vi "Process.vi"(0 "reference in":refnum<class "Tester.lvclass">, 5 "error in (no error)":errorcluster) -> (14 "reference out":refnum<class "Tester.lvclass">, 19 "error out":errorcluster)   [LabVIEW 2018, in "Tester.lvclass"]
uses:
  Tester.lvclass
  <vilib>/Utility/miscctls.llb/LVRowAndColumnUnsignedTypeDef.ctl
  controls/LR Mode.ctl
  Reporter_class/Reporter.lvclass
  BKP-911x Power Supply_class/BKP-911x Power Supply.lvclass
  NI-DAQmx_class/NI-DAQmx.lvclass
  BKP-891 LCR Meter_class/BKP-891 LCR Meter.lvclass
panel:
  out "Step Number":i32
  in  "Load Test":bool
  in  "Stop Test":bool
  in  "Start Test":bool
  out "Loaded Test Profile Path":path
  out "Loaded Test Profile":i32(listbox)
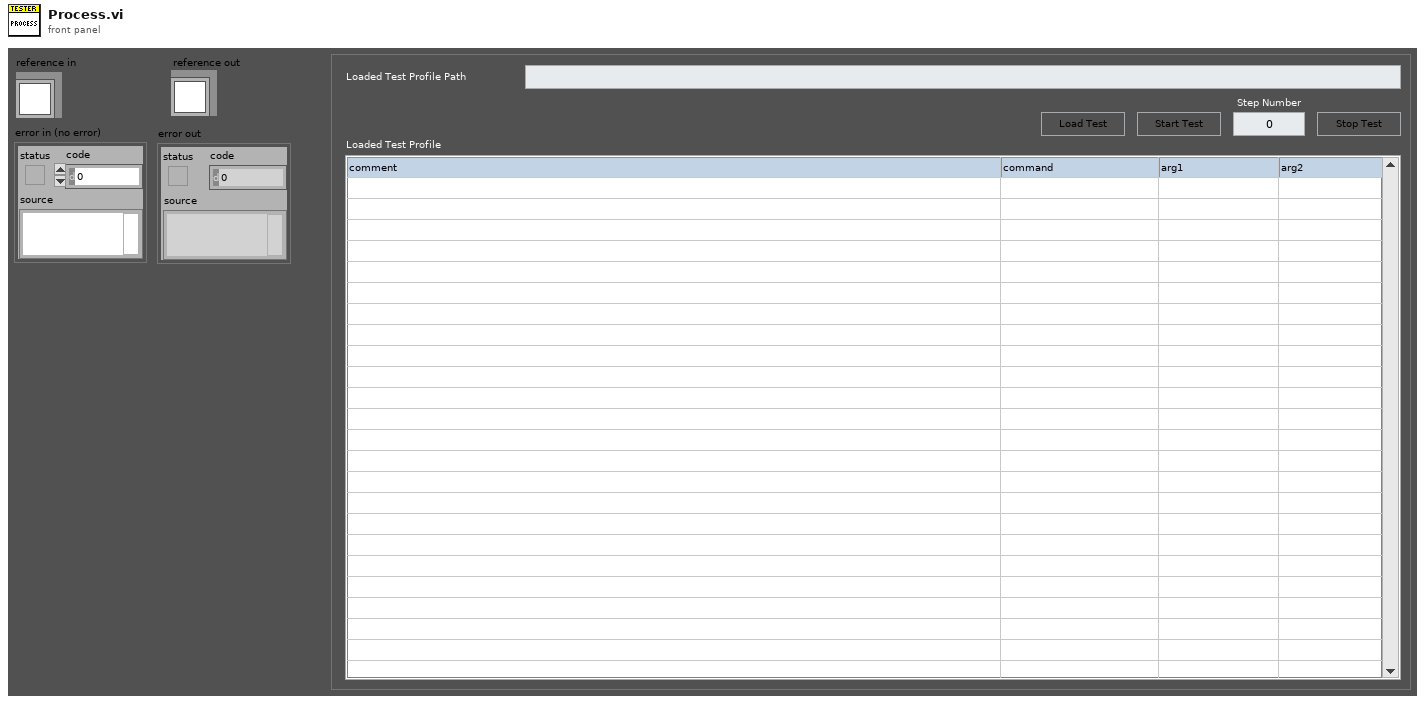
[diagram p1: front panel]
types:
  T1 = cluster{"Event":refnum<event-registration>, "Command":string, "Data":variant, "Testing?":bool, "Loaded Test Steps":string[][], "Args":variant, "Test Step Index":i32, "Step Comment":string}
  T2 = enum8{"Enabled", "Disabled", "Disabled and Grayed Out"}
  T3 = typedef "LVRowAndColumnUnsignedTypeDef.ctl" = cluster{"Row":u32, "Column":u32}
  T4 = typedef "LR Mode.ctl" = enum16{"R - Resistance", "L - Inductance"}
  T5 = typedef "Tester.lvclass/ObjectAttributes.ctl" = cluster{"LCR":refnum<class "BKP-891 LCR Meter.lvclass">, "PSU":refnum<class "BKP-911x Power Supply.lvclass">, "NI-DAQmx":refnum<class "NI-DAQmx.lvclass">, "Reporter":refnum<class "Reporter.lvclass">}
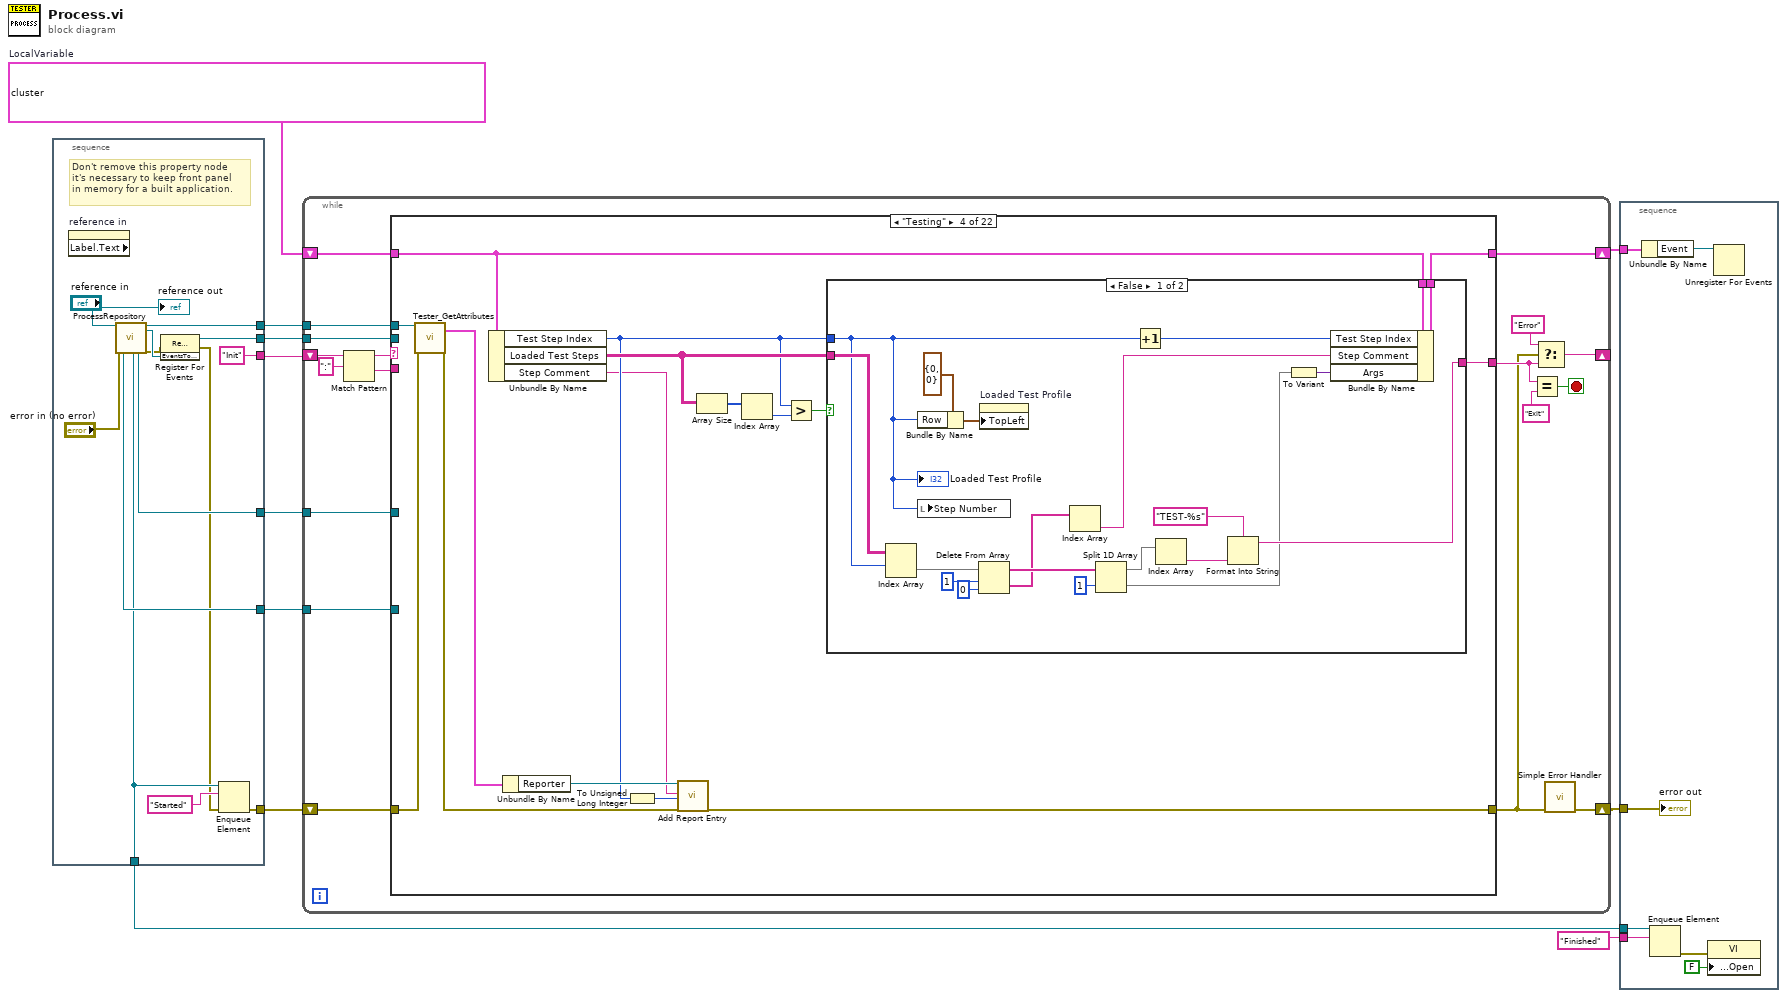
[diagram p0: block diagram]
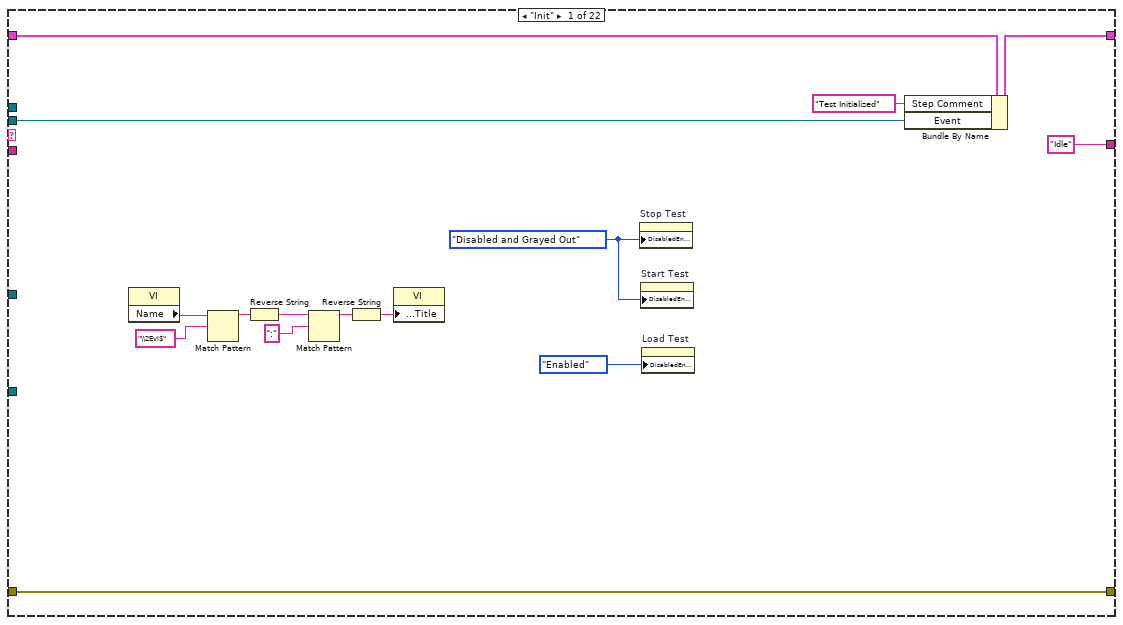
[diagram p2: hidden frame]
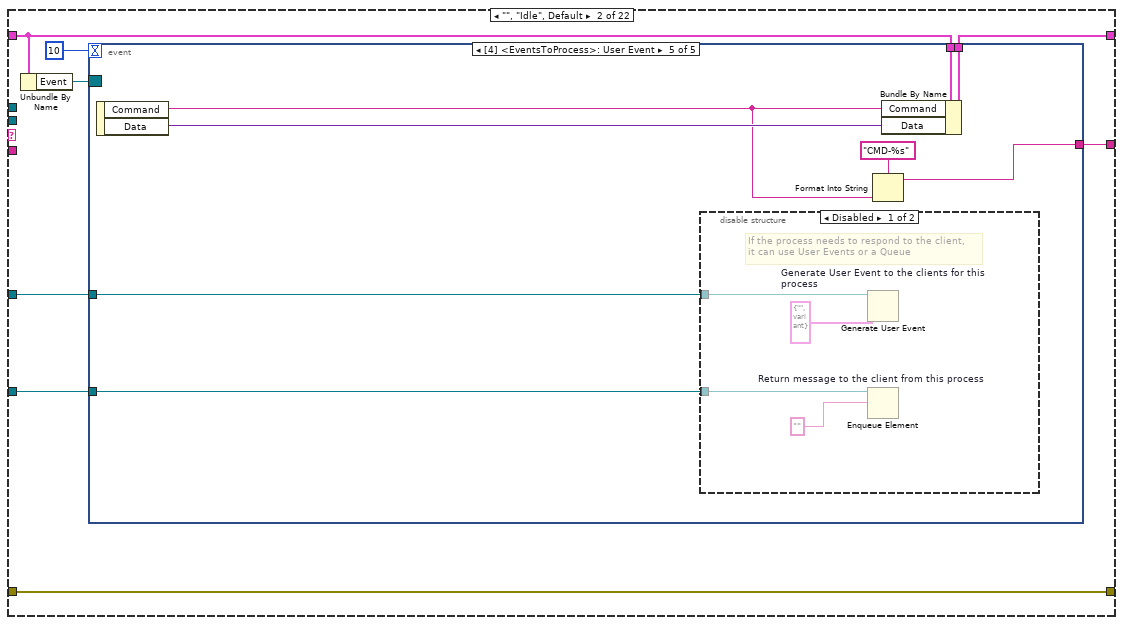
[diagram p3: hidden frame]
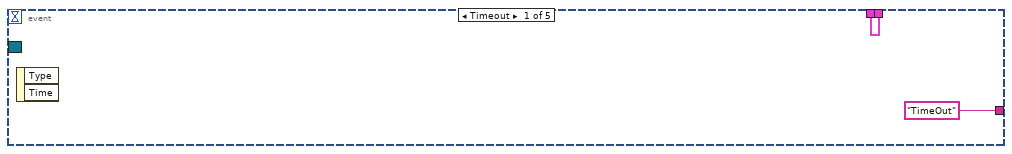
[diagram p4: hidden frame]
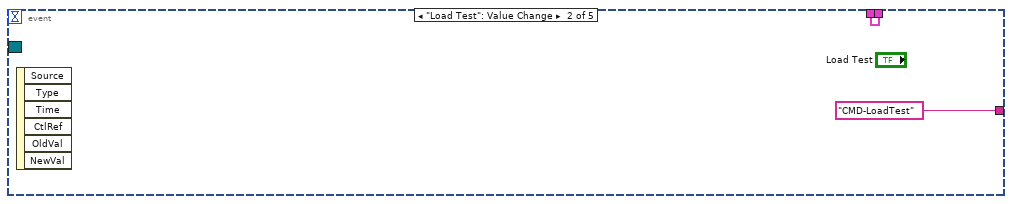
[diagram p5: hidden frame]
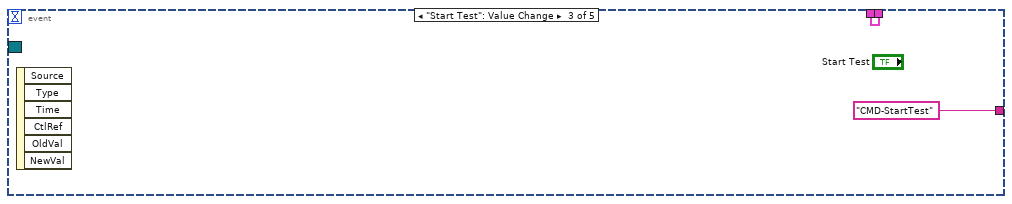
[diagram p6: hidden frame]
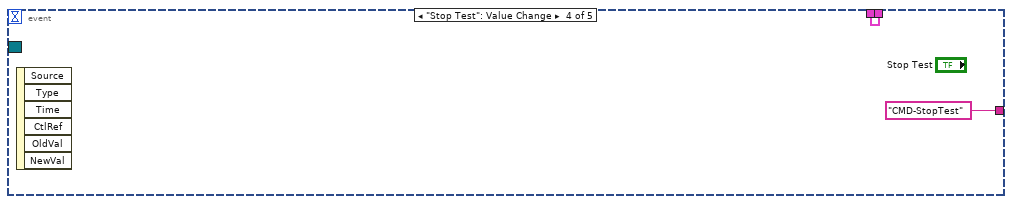
[diagram p7: hidden frame]
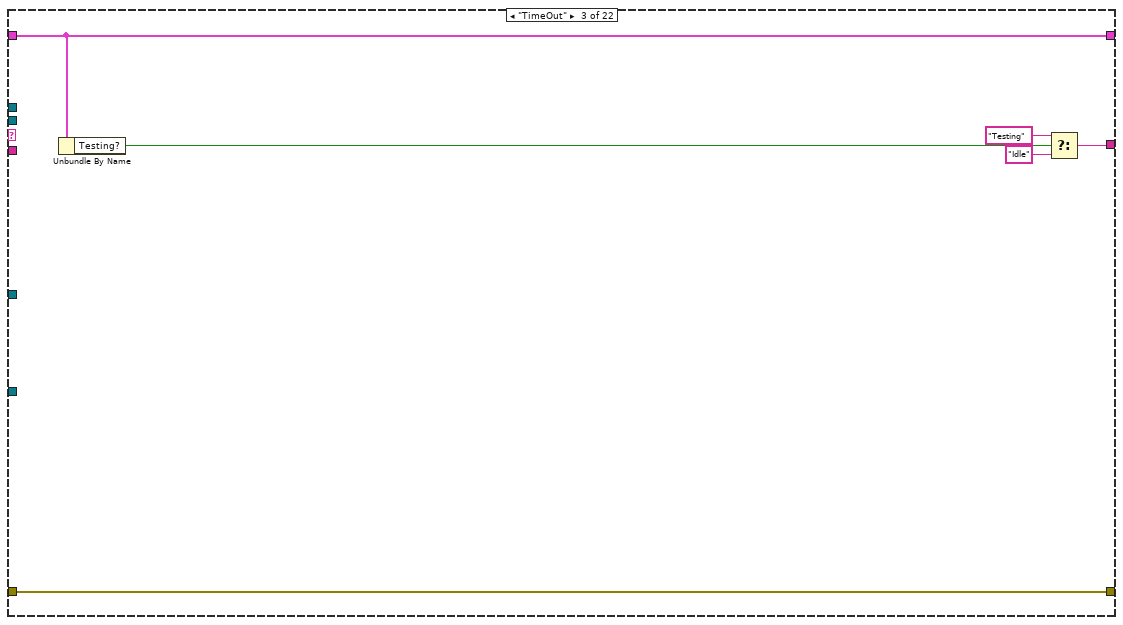
[diagram p9: hidden frame]
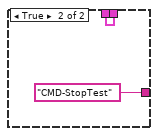
[diagram p10: hidden frame]
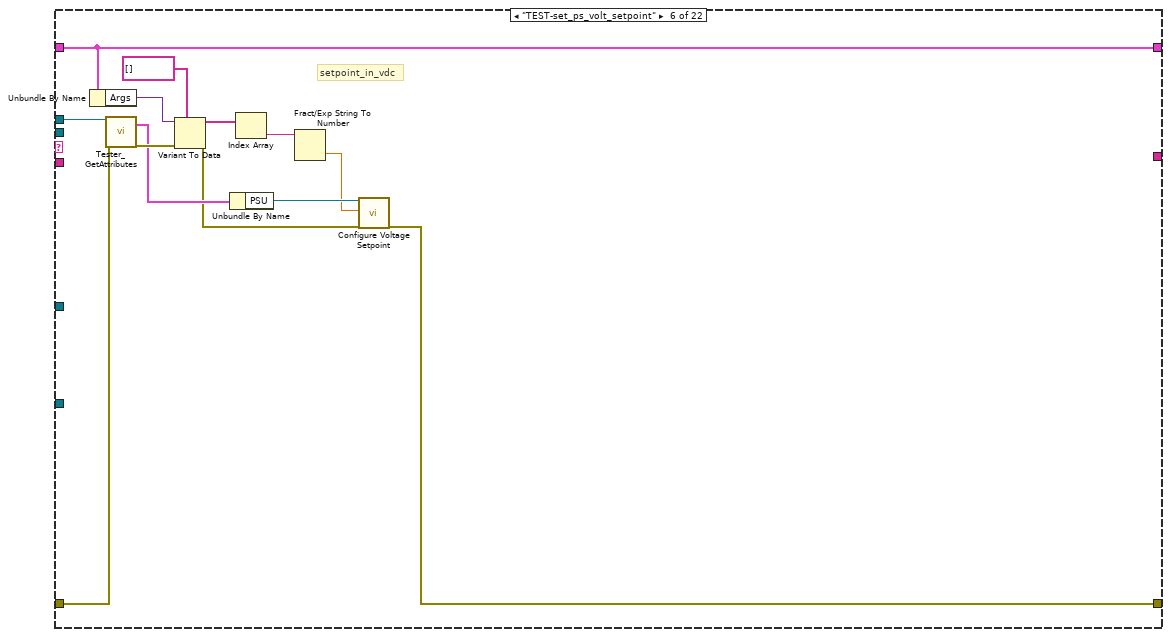
[diagram p12: hidden frame]
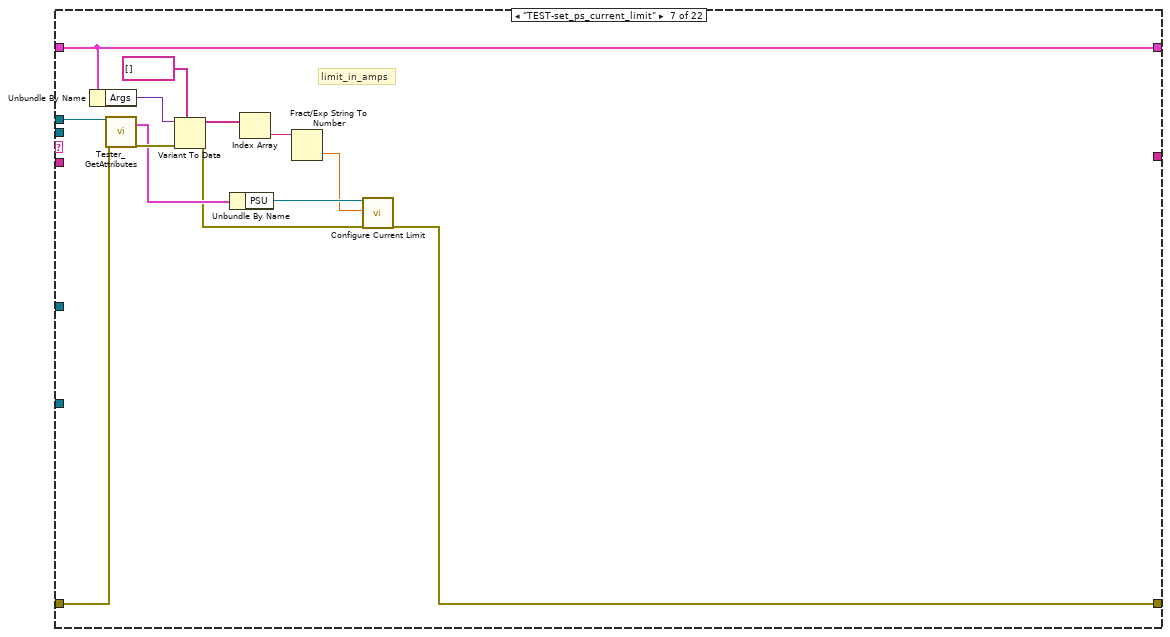
[diagram p13: hidden frame]
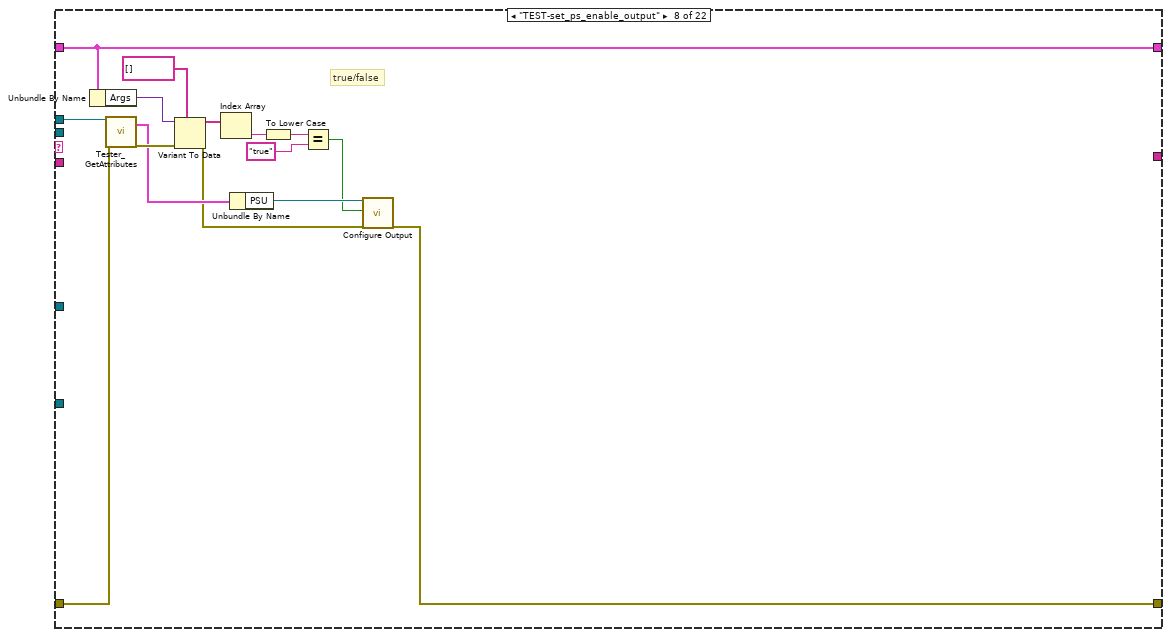
[diagram p14: hidden frame]
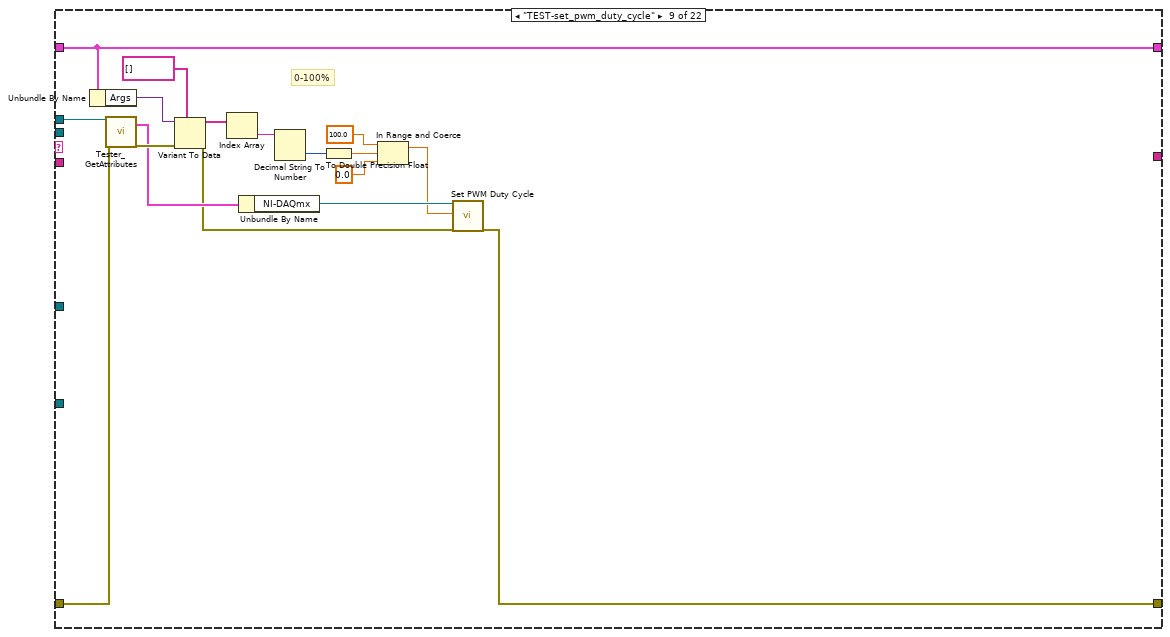
[diagram p15: hidden frame]
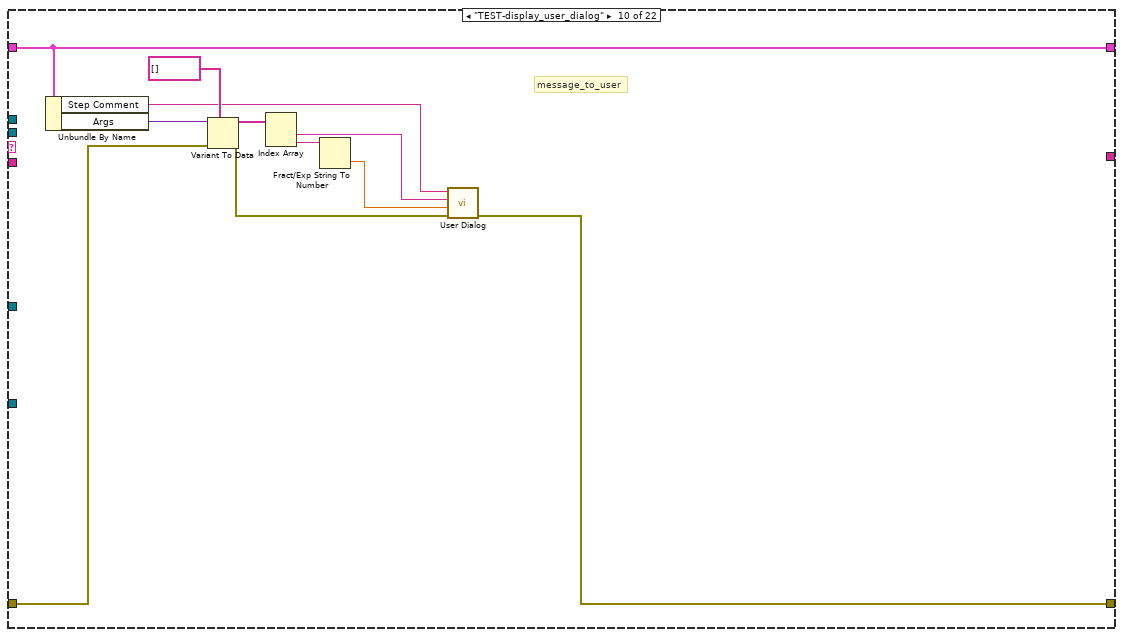
[diagram p16: hidden frame]
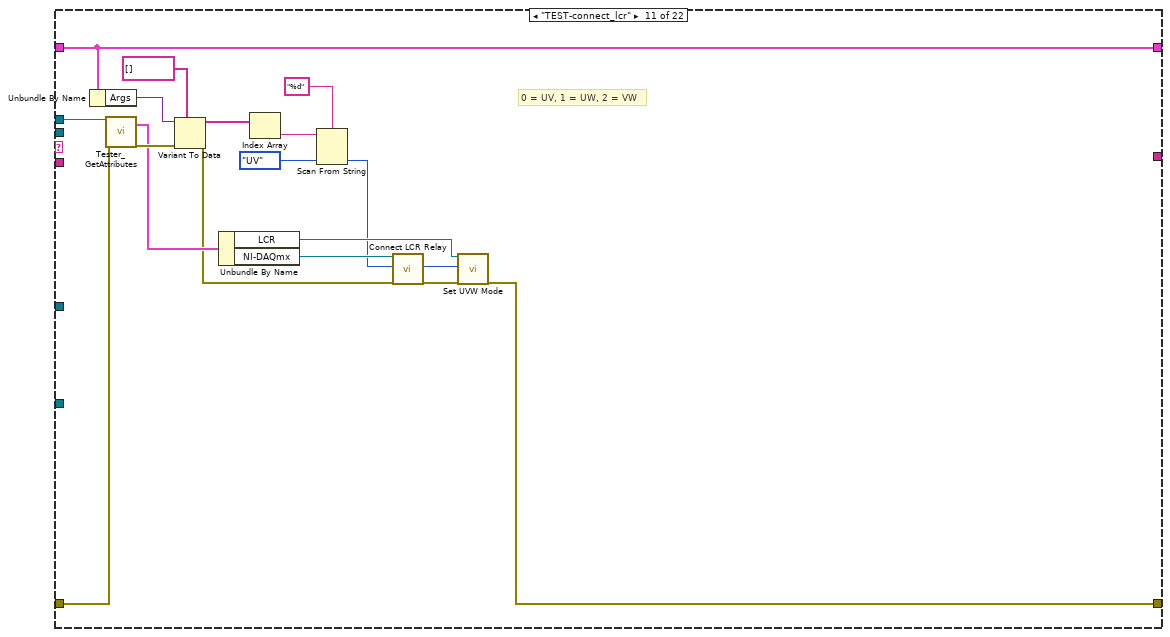
[diagram p17: hidden frame]
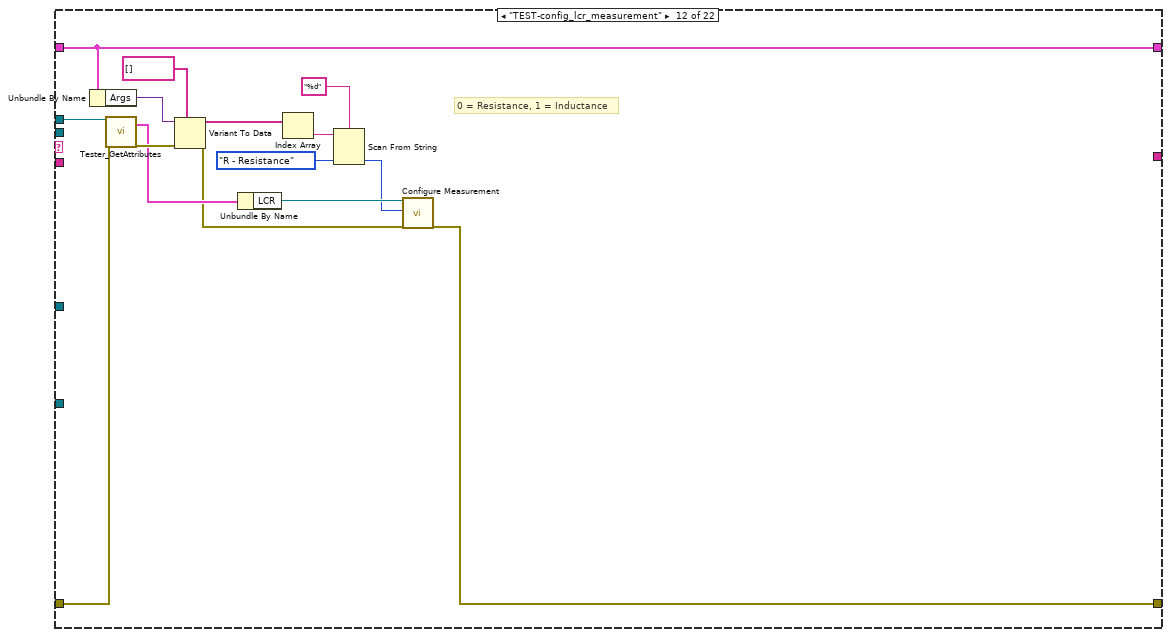
[diagram p18: hidden frame]
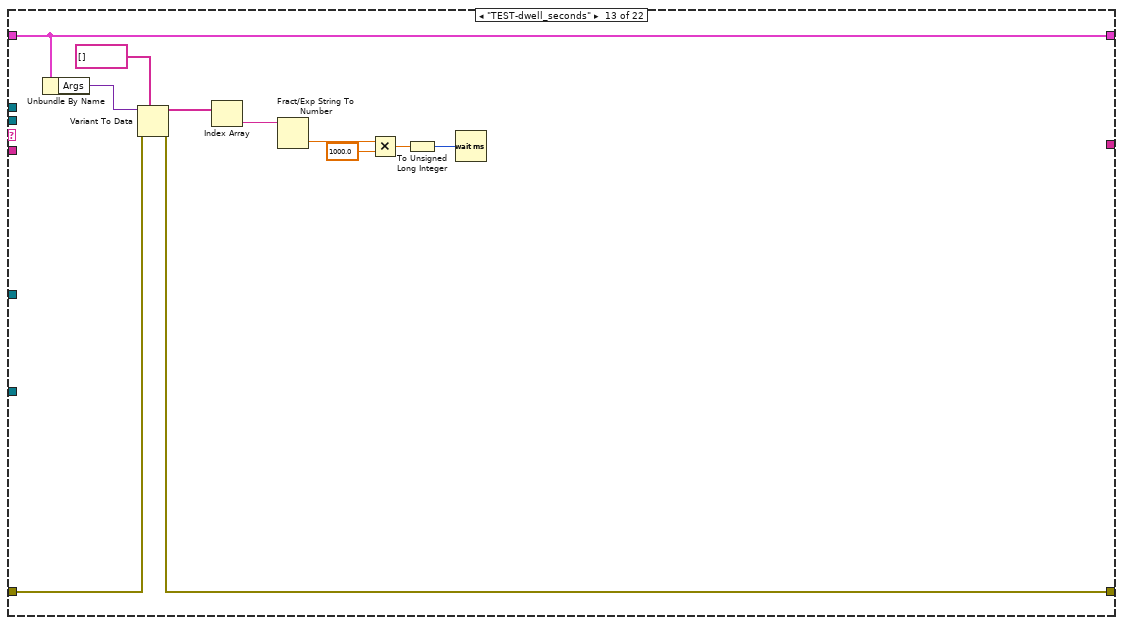
[diagram p19: hidden frame]
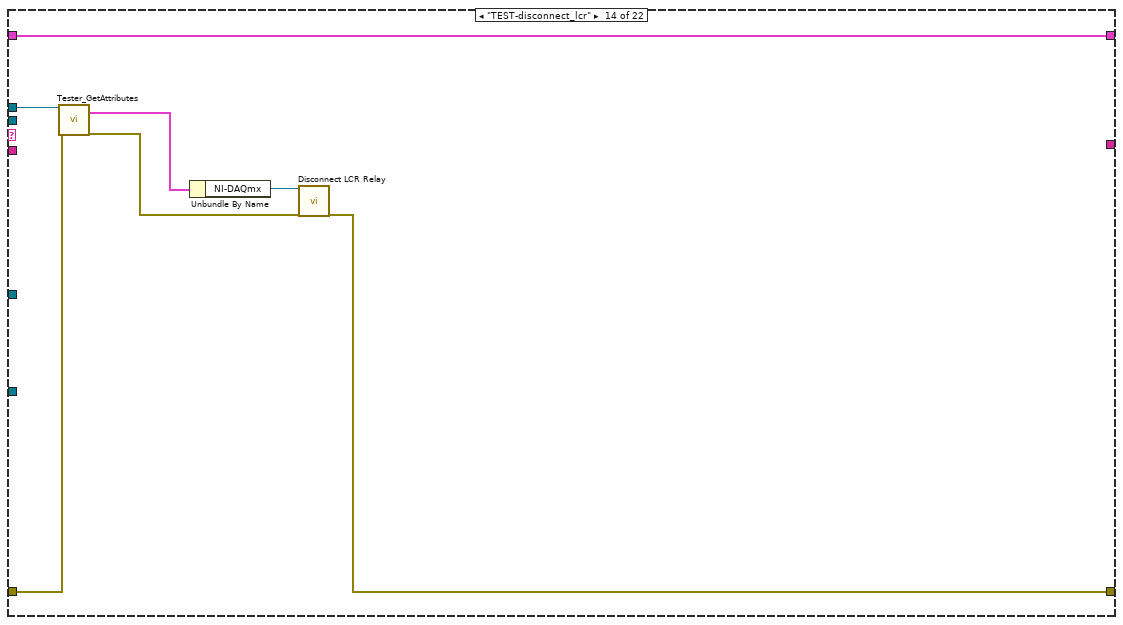
[diagram p20: hidden frame]
diagram:
  w1 = T1 {"Event"=refnum, "Command"="", "Data"=variant, "Testing?"=FALSE, "Loaded Test Steps"=[], "Args"=variant, "Test Step Index"=0, "Step Comment"=""}  # LocalVariable
  n1 = stacked-sequence {
    tunnel: [w17] -> w11
    tunnel: [w24] -> w9
    tunnel: [w14] -> w8
    tunnel: [w18] -> w7
    tunnel: ["Init"] -> w6
    tunnel: [w20] -> w4
    tunnel: [w19] -> w3
    frame #0 {
      # "Don't remove this property node\nit's necessary to keep front panel\nin memory for a built application."
      n2 = property on="reference in" class="LVClassControl (strict)" props=["Label", "Text"]() -> ()  [unwired: 2 in, 3 out]
      n3 = call "ProcessRepository.vi"("reference in"="reference in", "error in (no error)"="error in (no error)") -> ("QueueFromProcess"=w19:refnum<queue>, "ProcessSyncQueue"=w18:refnum<queue>, "EventFromProcess"=w20:refnum<user-event>, "reference out"=w24:refnum<class "Tester.lvclass">, "EventsToProcess"=w15:refnum<user-event>, "error out"=w13:errorcluster)  [unwired: 10 in, 2 out]
      n4 = register-events(error in=w13, w15) -> (reference out=w14:refnum<event-registration>, error out=w12:errorcluster)  [unwired: 1 in]
      n5 = Enqueue Element(queue=w18, element="Started", error in (no error)=w12) -> (error out=w17:errorcluster)  [unwired: 1 in, 2 out]
      "reference out" <- "reference in"
    }
  }
  n6 = while {
    shift-right: [w25] -> w10
    shift-left: w11 -> [w40]
    tunnel: w9 -> [w41]
    tunnel: w8 -> [w42]
    shift-right: [w34] -> _
    shift-left: w6 -> [w38]
    shift-right: [w30] -> w5
    shift-left: w1 -> [w29]
    tunnel: w4 -> [w28]
    tunnel: w3 -> [w27]
    stop <- w31 stop-if-true
    n7 = Match Pattern(string=w38, regular expression=":") -> (before substring=w37:string, after substring=w36:string)  [unwired: 1 in, 2 out]
    n8 = case shown="\"Testing\"" w37 {
      tunnel: w40 -> [w56 w61 w91 w99 w131 w143 w156 w171 w188 w200 w216 w231 w243 w249 w256 w259 w261 _ w306 w331 w350 w353]
      tunnel: [w56 w61 w91 w95 w131 w132 w145 w160 w180 w193 w203 w221 w238 w244 w251 w259 w261 w262 w301 w330 w350 w353] -> w26
      tunnel: w42 -> [w47 _ _ _ _ _ _ _ _ _ _ _ _ _ _ _ _ _ _ _ _ _]
      tunnel: w41 -> [_ _ _ w100 _ w144 w157 w172 w189 _ w217 w232 _ w250 w257 _ _ _ w305 w332 _ _]
      tunnel: w36 -> [_ _ _ _ _ _ _ _ _ _ _ _ _ _ _ _ _ _ _ _ _ _]
      tunnel: ["Idle" ("t") w65 w86 w105 _ _ _ _ _ _ _ _ _ _ _ _ _ _ w315 w335 _ "Exit" ("y")] -> w33
      tunnel: [w57 w64 w90 w106 w130 w142 w155 w170 w187 w199 w215 w230 w242 w248 w255 w258 w260 w263 w314 w336 w349 w351] -> w30
      tunnel: w29 -> [w46 w58 w90 w107 w130 w142 w155 w170 w187 w199 w215 w230 w242 w248 w255 w258 w260 w264 w313 w334 w349 w351]
      tunnel: w28 -> [_ w60 _ _ _ _ _ _ _ _ _ _ _ _ _ _ _ _ _ _ _ _]
      tunnel: w27 -> [_ w59 _ _ _ _ _ _ _ _ _ _ _ _ _ _ _ _ _ _ _ _]
      frame "Init" {
        w44 = T2."Disabled and Grayed Out" ("Disabled")
        n9 = property class="VI"() -> ("Name"=w54:string)  [unwired: 2 in, 2 out]
        n10 = Match Pattern(string=w54, regular expression="\\2Evi$") -> (before substring=w52:string)  [unwired: 1 in, 3 out]
        n11 = Reverse String(1:w52) -> (0:w51:string)
        n12 = Match Pattern(string=w51, regular expression=":") -> (before substring=w49:string)  [unwired: 1 in, 3 out]
        n13 = Reverse String(1:w49) -> (0:w48:string)
        n14 = property class="VI"("Front Panel.Title"=w48) -> ()  [unwired: 2 in, 2 out]
        n15 = property on="Stop Test" class="Bool"("DisabledEnum"=w44) -> ()  [unwired: 2 in, 2 out]
        n16 = property on="Start Test" class="Bool"("DisabledEnum"=w44) -> ()  [unwired: 2 in, 2 out]
        n17 = property on="Load Test" class="Bool"("DisabledEnum"=T2."Enabled" ("Disabled")) -> ()  [unwired: 2 in, 2 out]
        n18 = Bundle By Name(cluster=w46, "Step Comment"="Test Initialized", "Event"=w47) -> (w57:T1)
      }
      frame "", "Idle", Default {
        n19 = Unbundle By Name(w58) -> ("Event"=w63:refnum<event-registration>)
        n20 = event shown="[4] <EventsToProcess>: User Event" {
          selector: w63 -> [_ _ _ _ _]
          dyn-events: _ -> [_ _ _ _ _]
          timeout: 10 -> [_ _ _ _ _]
          tunnel: ["TimeOut" ("t") "CMD-LoadTest" ("t") "CMD-StartTest" ("t") "CMD-StopTest" ("t") w77] -> w65
          tunnel: w58 -> [w66 w69 w71 w73 w81]
          tunnel: [w66 w69 w71 w73 w80] -> w64
          tunnel: w60 -> [_ _ _ _ w75]
          tunnel: w59 -> [_ _ _ _ w74]
          event Timeout {
            n21 = event-data() -> ()  [unwired: 1 in, 2 out]
          }
          event "Load Test": Value Change {
            n22 = event-data() -> ()  [unwired: 1 in, 6 out]
          }
          event "Start Test": Value Change {
            n23 = event-data() -> ()  [unwired: 1 in, 6 out]
          }
          event "Stop Test": Value Change {
            n24 = event-data() -> ()  [unwired: 1 in, 6 out]
          }
          event User Event {
            n25 = event-data() -> ("Command"=w76:string, "Data"=w79:variant)  [unwired: 1 in]
            n26 = disable-structure shown="Disabled" {
              disable-tunnel: w75 -> [w85 _]
              disable-tunnel: w74 -> [w84 _]
              frame Disabled {
                # "If the process needs to respond to the client,\nit can use User Events or a Queue"
                n27 = Generate User Event "Generate User Event to the clients for this process"(user event=w85, event data cluster=cluster{"Command":string, "Data":variant} {"Command"="", "Data"=variant} ("event data")) -> ()  [unwired: 2 in, 2 out]
                n28 = Enqueue Element "Return message to the client from this process"(queue=w84, element="") -> ()  [unwired: 2 in, 3 out]
              }
              frame Enabled {
              }
            }
            n29 = Format Into String(format string="CMD-%s", w76) -> (resulting string=w77:string)  [unwired: 2 in, 1 out]
            n30 = Bundle By Name(cluster=w81, "Command"=w76, "Data"=w79) -> (w80:T1)
          }
        }
      }
      frame "TimeOut" {
        n31 = Unbundle By Name(w90) -> ("Testing?"=w89:bool)
        n32 = Select(t="Testing", s=w89, f="Idle" ("t")) -> (s? t:f=w86:string)
      }
      frame "Testing" {
        n33 = call "Tester_GetAttributes.vi"("reference in"=w100, "error in (no error)"=w99) -> ("Data"=w98:T5, "error out"=w96:errorcluster)  [unwired: 14 in, 2 out]
        n34 = Unbundle By Name(w107) -> ("Test Step Index"=w94:i32, "Loaded Test Steps"=w104:string[][], "Step Comment"=w92:string)
        n35 = Unbundle By Name(w98) -> ("Reporter"=w97:refnum<class "Reporter.lvclass">)
        n36 = To Unsigned Long Integer(number=w94) -> (unsigned 32bit integer=w93:u32)
        n37 = call-dynamic "Add Report Entry.vi"("reference in"=w97, "comment"=w92, "step_index"=w93, "error in (no error)"=w96) -> ("error out"=w95:errorcluster)  [unwired: 14 in, 1 out]
        n38 = Array Size(array=w104) -> (size(s)=w103:i32[])
        n39 = Index Array(array=w103) -> (element=w102:i32)  [unwired: 1 in]
        n40 = Greater?(x=w94, y=w102) -> (0:w101:bool)
        n41 = case shown="False" w101 {
          tunnel: w107 -> [w127 w129]
          tunnel: [w126 w129] -> w106
          tunnel: w104 -> [w124 _]
          tunnel: w94 -> [w109 _]
          tunnel: [w115 "CMD-StopTest" ("y")] -> w105
          frame False {
            n42 = Index Array(array=w124, index (row)=w109) -> (element=w123:string[])  [unwired: 1 in]
            n43 = Bundle By Name(cluster=T3 {"Row"=0, "Column"=0} ("Top Left Visible Cell"), "Row"=w109) -> (w108:T3)
            n44 = local write "Step Number"(w109) -> ()
            n45 = Delete From Array(array=w123, length=1, index=0) -> (deleted portion=w112:string[], array with subset deleted=w120:string[])
            n46 = property on="Loaded Test Profile" class="MCListbox (strict)"("TopLeft"=w108) -> ()  [unwired: 2 in, 2 out]
            n47 = Index Array(array=w112) -> (element=w111:string)  [unwired: 1 in]
            n48 = Split 1D Array(array=w120, index=1) -> (first subarray=w118:string[], second subarray=w114:string[])
            n49 = Increment(x=w109) -> (x+1=w125:i32)
            n50 = Index Array(array=w118) -> (element=w116:string)  [unwired: 1 in]
            n51 = Format Into String(format string="TEST-%s", w116) -> (resulting string=w115:string)  [unwired: 2 in, 1 out]
            n52 = To Variant(anything=w114) -> (Variant=w113:variant)
            n53 = Bundle By Name(cluster=w127, "Test Step Index"=w125, "Step Comment"=w111, "Args"=w113) -> (w126:T1)
            "Loaded Test Profile" <- w109
          }
          frame True {
          }
        }
      }
      frame "---- TEST METHODS START ----" {
        # "read arguments from variant in shift register"
      }
      frame "TEST-set_ps_volt_setpoint" {
        # "setpoint_in_vdc"
        n54 = Unbundle By Name(w142) -> ("Args"=w140:variant)
        n55 = call "Tester_GetAttributes.vi"("reference in"=w144, "error in (no error)"=w143) -> ("Data"=w138:T5, "error out"=w141:errorcluster)  [unwired: 14 in, 2 out]
        n56 = Variant To Data(error in=w141, type=string[] [], Variant=w140) -> (data=w137:string[], error out=w133:errorcluster)
        n57 = Unbundle By Name(w138) -> ("PSU"=w135:refnum<class "BKP-911x Power Supply.lvclass">)
        n58 = Index Array(array=w137) -> (element=w136:string)  [unwired: 1 in]
        n59 = Fract/Exp String To Number(string=w136) -> (number=w134:dbl)  [unwired: 3 in, 1 out]
        n60 = call-dynamic "Configure Voltage Setpoint.vi"("reference in"=w135, "Voltage Setpoint (V)"=w134, "error in (no error)"=w133) -> ("error out"=w132:errorcluster)  [unwired: 15 in, 1 out]
      }
      frame "TEST-set_ps_current_limit" {
        # "limit_in_amps"
        n61 = Unbundle By Name(w155) -> ("Args"=w153:variant)
        n62 = call "Tester_GetAttributes.vi"("reference in"=w157, "error in (no error)"=w156) -> ("Data"=w151:T5, "error out"=w154:errorcluster)  [unwired: 14 in, 2 out]
        n63 = Variant To Data(error in=w154, type=string[] [], Variant=w153) -> (data=w150:string[], error out=w146:errorcluster)
        n64 = Unbundle By Name(w151) -> ("PSU"=w148:refnum<class "BKP-911x Power Supply.lvclass">)
        n65 = Index Array(array=w150) -> (element=w149:string)  [unwired: 1 in]
        n66 = Fract/Exp String To Number(string=w149) -> (number=w147:dbl)  [unwired: 3 in, 1 out]
        n67 = call-dynamic "Configure Current Limit.vi"("reference in"=w148, "Current Limit (0.0 A)"=w147, "error in (no error)"=w146) -> ("error out"=w145:errorcluster)  [unwired: 15 in, 1 out]
      }
      frame "TEST-set_ps_enable_output" {
        # "true/false"
        n68 = Unbundle By Name(w170) -> ("Args"=w168:variant)
        n69 = call "Tester_GetAttributes.vi"("reference in"=w172, "error in (no error)"=w171) -> ("Data"=w166:T5, "error out"=w169:errorcluster)  [unwired: 14 in, 2 out]
        n70 = Variant To Data(error in=w169, type=string[] [], Variant=w168) -> (data=w165:string[], error out=w161:errorcluster)
        n71 = Index Array(array=w165) -> (element=w159:string)  [unwired: 1 in]
        n72 = Unbundle By Name(w166) -> ("PSU"=w163:refnum<class "BKP-911x Power Supply.lvclass">)
        n73 = To Lower Case(string=w159) -> (all lower case string=w158:string)
        n74 = Equal?(x=w158, y="true") -> (x = y?=w162:bool)
        n75 = call-dynamic "Configure Output.vi"("reference in"=w163, "Enable Output (T: Enable)"=w162, "error in (no error)"=w161) -> ("error out"=w160:errorcluster)  [unwired: 15 in, 1 out]
      }
      frame "TEST-set_pwm_duty_cycle" {
        # "0-100%"
        n76 = Unbundle By Name(w187) -> ("Args"=w185:variant)
        n77 = call "Tester_GetAttributes.vi"("reference in"=w189, "error in (no error)"=w188) -> ("Data"=w183:T5, "error out"=w186:errorcluster)  [unwired: 14 in, 2 out]
        n78 = Variant To Data(error in=w186, type=string[] [], Variant=w185) -> (data=w179:string[], error out=w181:errorcluster)
        n79 = Index Array(array=w179) -> (element=w178:string)  [unwired: 1 in]
        n80 = Unbundle By Name(w183) -> ("NI-DAQmx"=w182:refnum<class "NI-DAQmx.lvclass">)
        n81 = Decimal String To Number(string=w178) -> (number=w177:i32)  [unwired: 2 in, 1 out]
        n82 = To Double Precision Float(number=w177) -> (double precision float=w176:dbl)
        n83 = In Range and Coerce(upper limit=100.0, x=w176, lower limit=0.0) -> (coerced(x)=w173:dbl)  [unwired: 1 out]
        n84 = call-dynamic "Set PWM Duty Cycle.vi"("reference in"=w182, "PWM Duty Cycle (%)"=w173, "error in (no error)"=w181) -> ("error out"=w180:errorcluster)  [unwired: 15 in, 1 out]
      }
      frame "TEST-display_user_dialog" {
        # "message_to_user"
        n85 = Unbundle By Name(w199) -> ("Step Comment"=w190:string, "Args"=w198:variant)
        n86 = Variant To Data(error in=w200, type=string[] [], Variant=w198) -> (data=w196:string[], error out=w194:errorcluster)
        n87 = Index Array(array=w196) -> (element #1=w195:string, element #2=w192:string)  [unwired: 2 in]
        n88 = Fract/Exp String To Number(string=w192) -> (number=w191:dbl)  [unwired: 3 in, 1 out]
        n89 = call "User Dialog.vi"("error in (no error)"=w194, "Timeout (seconds)"=w191, "Message"=w195, "Title"=w190) -> ("error out"=w193:errorcluster)  [unwired: 7 in]
      }
      frame "TEST-connect_lcr" {
        # "0 = UV, 1 = UW, 2 = VW"
        n90 = Unbundle By Name(w215) -> ("Args"=w213:variant)
        n91 = call "Tester_GetAttributes.vi"("reference in"=w217, "error in (no error)"=w216) -> ("Data"=w211:T5, "error out"=w214:errorcluster)  [unwired: 14 in, 2 out]
        n92 = Variant To Data(error in=w214, type=string[] [], Variant=w213) -> (data=w208:string[], error out=w209:errorcluster)
        n93 = Unbundle By Name(w211) -> ("LCR"=w202:refnum<class "BKP-891 LCR Meter.lvclass">, "NI-DAQmx"=w210:refnum<class "NI-DAQmx.lvclass">)
        n94 = Index Array(array=w208) -> (element=w206:string)  [unwired: 1 in]
        n95 = Scan From String(format string="%d", input string=w206, default 1=enum16{"UV", "UW", "VW"}."UV" ("Relay Mode")) -> (output 1=w201:enum16{"UV", "UW", "VW"})  [unwired: 2 in, 3 out]
        n96 = call-dynamic "Connect LCR Relay.vi"("reference in"=w210, "Relay Mode"=w201, "error in (no error)"=w209) -> ("error out"=w204:errorcluster)  [unwired: 15 in, 1 out]
        n97 = call-dynamic "Set UVW Mode.vi"("reference in"=w202, "UVW Mode"=w201, "error in (no error)"=w204) -> ("error out"=w203:errorcluster)  [unwired: 15 in, 1 out]
      }
      frame "TEST-config_lcr_measurement" {
        # "0 = Resistance, 1 = Inductance"
        n98 = Unbundle By Name(w230) -> ("Args"=w228:variant)
        n99 = call "Tester_GetAttributes.vi"("reference in"=w232, "error in (no error)"=w231) -> ("Data"=w226:T5, "error out"=w229:errorcluster)  [unwired: 14 in, 2 out]
        n100 = Variant To Data(error in=w229, type=string[] [], Variant=w228) -> (data=w225:string[], error out=w222:errorcluster)
        n101 = Unbundle By Name(w226) -> ("LCR"=w220:refnum<class "BKP-891 LCR Meter.lvclass">)
        n102 = Index Array(array=w225) -> (element=w224:string)  [unwired: 1 in]
        n103 = Scan From String(format string="%d", input string=w224, default 1=LR_Mode."R - Resistance" ("LR Mode")) -> (output 1=w218:T4)  [unwired: 2 in, 3 out]
        n104 = call-dynamic "Configure Measurement.vi"("reference in"=w220, "LR Mode"=w218, "error in (no error)"=w222) -> ("error out"=w221:errorcluster)  [unwired: 15 in, 1 out]
      }
      frame "TEST-dwell_seconds" {
        n105 = Unbundle By Name(w242) -> ("Args"=w241:variant)
        n106 = Variant To Data(error in=w243, type=string[] [], Variant=w241) -> (data=w239:string[], error out=w238:errorcluster)
        n107 = Index Array(array=w239) -> (element=w237:string)  [unwired: 1 in]
        n108 = Fract/Exp String To Number(string=w237) -> (number=w236:dbl)  [unwired: 3 in, 1 out]
        n109 = Multiply(x=w236, y=1000.0) -> (x*y=w234:dbl)
        n110 = To Unsigned Long Integer(number=w234) -> (unsigned 32bit integer=w233:u32)
        n111 = Wait (ms)(milliseconds to wait=w233) -> ()  [unwired: 1 out]
      }
      frame "TEST-disconnect_lcr" {
        n112 = call "Tester_GetAttributes.vi"("reference in"=w250, "error in (no error)"=w249) -> ("Data"=w247:T5, "error out"=w245:errorcluster)  [unwired: 14 in, 2 out]
        n113 = Unbundle By Name(w247) -> ("NI-DAQmx"=w246:refnum<class "NI-DAQmx.lvclass">)
        n114 = call-dynamic "Disconnect LCR Relay.vi"("reference in"=w246, "error in (no error)"=w245) -> ("error out"=w244:errorcluster)  [unwired: 16 in, 1 out]
      }
      frame "TEST-tare_lcr" {
        n115 = call "Tester_GetAttributes.vi"("reference in"=w257, "error in (no error)"=w256) -> ("Data"=w254:T5, "error out"=w252:errorcluster)  [unwired: 14 in, 2 out]
        n116 = Unbundle By Name(w254) -> ("LCR"=w253:refnum<class "BKP-891 LCR Meter.lvclass">)
        n117 = call-dynamic "Set Tare Offset.vi"("reference in"=w253, "error in (no error)"=w252) -> ("error out"=w251:errorcluster)  [unwired: 16 in, 1 out]
      }
      frame "---- TEST METHODS END ----" {
      }
      frame "---- COMMANDS START----" {
      }
      frame "CMD-LoadTest" {
        n118 = call "Get File Paths.vi"() -> ("Test Profiles Directory"=w273:path)  [unwired: 10 in, 1 out]
        n119 = call "File Dialog"("start path"=w273, "prompt"="Select a test profile (csv) to load...", "button label"="Load Test", "pattern (all files)"="*.csv", "pattern label"="Comma Separated Values") -> ("selected path"=w267:path, "cancelled"=w268:bool, "error out"=w266:errorcluster)  [unwired: 7 in, 1 out]
        n120 = call <vilib>:"Clear Errors.vi"("error in (no error)"=w266) -> ("error out"=w265:errorcluster)  [unwired: 5 in, 1 out]
        n121 = case shown="False" w268 {
          tunnel: w267 -> [w295 _]
          tunnel: w265 -> [w296 w299]
          tunnel: w264 -> [w298 w300]
          tunnel: [w297 w300] -> w263
          tunnel: [w277 w299] -> w262
          frame False {
            # "remove header row"
            n122 = Open/Create/Replace File(file path (use dialog)=w295, error in=w296, access (0:read/write)=enum16{"read/write", "read-only", "write-only"}."read-only") -> (refnum out=w293:refnum<file>, error out=w292:errorcluster)  [unwired: 3 in, 1 out]
            n123 = Read from Text File(file (use dialog)=w293, error in=w292) -> (refnum out=w290:refnum<file>, text=w289:string, error out=w291:errorcluster)  [unwired: 2 in, 1 out]
            n124 = Close File(refnum=w290, error in=w291) -> (path=→"Loaded Test Profile Path":path, error out=w281:errorcluster)
            n125 = Spreadsheet String To Array(delimiter (Tab)=",", format string="%s", spreadsheet string=w289, array type (2D Dbl)=string[][] [] ("Test Steps")) -> (array=w284:string[][])
            n126 = Delete From Array(array=w284, length=1, index (row)=0) -> (array with subset deleted=w275:string[][])  [unwired: 1 in, 1 out]
            n127 = property on="Start Test" class="Bool"(error in=w281, "DisabledEnum"=T2."Enabled" ("Disabled")) -> (error out=w279:errorcluster)  [unwired: 1 in, 1 out]
            n128 = property on="Loaded Test Profile" class="MCListbox (strict)"("ItemNames"=w275) -> ()  [unwired: 2 in, 2 out]
            n129 = property on="Stop Test" class="Bool"(error in=w279, "DisabledEnum"=T2."Disabled and Grayed Out" ("Disabled")) -> (error out=w277:errorcluster)  [unwired: 1 in, 1 out]
            n130 = Bundle By Name(cluster=w298, "Test Step Index"=0, "Loaded Test Steps"=w275) -> (w297:T1)
            "Step Number" <- 0 ("Step Number")
          }
          frame True {
          }
        }
      }
      frame "CMD-StartTest" {
        # "verify test steps are loaded and that we are not already testing"
        n131 = call "Tester_GetAttributes.vi"("reference in"=w305, "error in (no error)"=w306) -> ("Data"=w303:T5, "error out"=w304:errorcluster)  [unwired: 14 in, 2 out]
        n132 = Unbundle By Name(w303) -> ("Reporter"=w302:refnum<class "Reporter.lvclass">)
        n133 = Unbundle By Name(w313) -> ("Loaded Test Steps"=w312:string[][], "Testing?"=w311:bool)
        n134 = Empty Array?(array=w312) -> (empty?=w308:bool)
        n135 = Not(x=w308) -> (.not. x?=w307:bool)
        n136 = Not(x=w311) -> (.not. x?=w310:bool)
        n137 = And(x=w307, y=w310) -> (x .and. y?=w309:bool)
        n138 = case shown="True" w309 {
          tunnel: ["Testing" ("t") _] -> w315
          tunnel: w313 -> [w322 w326]
          tunnel: [w321 w326] -> w314
          tunnel: w304 -> [w318 w325]
          tunnel: w302 -> [w317 _]
          tunnel: [w316 w325] -> w301
          frame True {
            w319 = T2."Disabled and Grayed Out" ("Disabled")
            n139 = call-dynamic "Open Report.vi"("reference in"=w317, "error in (no error)"=w318) -> ("error out"=w316:errorcluster)  [unwired: 16 in, 1 out]
            n140 = Bundle By Name(cluster=w322, "Testing?"=TRUE) -> (w321:T1)
            n141 = property on="Stop Test" class="Bool"("DisabledEnum"=T2."Enabled" ("Disabled")) -> ()  [unwired: 2 in, 2 out]
            n142 = property on="Start Test" class="Bool"("DisabledEnum"=w319) -> ()  [unwired: 2 in, 2 out]
            n143 = property on="Load Test" class="Bool"("DisabledEnum"=w319) -> ()  [unwired: 2 in, 2 out]
          }
          frame False {
          }
        }
      }
      frame "CMD-StopTest" {
        n144 = call "Tester_GetAttributes.vi"("reference in"=w332, "error in (no error)"=w331) -> ("Data"=w328:T5, "error out"=w329:errorcluster)  [unwired: 14 in, 2 out]
        n145 = Unbundle By Name(w328) -> ("Reporter"=w327:refnum<class "Reporter.lvclass">)
        n146 = Unbundle By Name(w334) -> ("Testing?"=w333:bool)
        n147 = case shown="True" w333 {
          tunnel: [_ "Idle" ("t")] -> w335
          tunnel: w334 -> [w338 w346]
          tunnel: [w338 w345] -> w336
          tunnel: [w337 w341] -> w330
          tunnel: w329 -> [w337 w342]
          tunnel: w327 -> [_ w340]
          frame False {
          }
          frame True {
            w343 = T2."Enabled" ("Disabled")
            n148 = call-dynamic "Close Report.vi"("reference in"=w340, "error in (no error)"=w342) -> ("error out"=w341:errorcluster)  [unwired: 16 in, 1 out]
            n149 = Bundle By Name(cluster=w346, "Testing?"=FALSE, "Step Comment"="Test Initialized") -> (w345:T1)
            n150 = property on="Stop Test" class="Bool"("DisabledEnum"=T2."Disabled and Grayed Out" ("Disabled")) -> ()  [unwired: 2 in, 2 out]
            n151 = property on="Start Test" class="Bool"("DisabledEnum"=w343) -> ()  [unwired: 2 in, 2 out]
            n152 = property on="Load Test" class="Bool"("DisabledEnum"=w343) -> ()  [unwired: 2 in, 2 out]
          }
        }
      }
      frame "----- COMMANDS END ----" {
      }
      frame "CMD-shutdown", "Error" {
      }
    }
    n153 = Equal?(x=w33, y="Exit") -> (x = y?=w31:bool)
    n154 = Select(t="Error", s=w26, f=w33) -> (s? t:f=w34:string)
    n155 = call <vilib>:"Simple Error Handler.vi"("error in (no error)"=w26) -> ("error out"=w25:errorcluster)  [unwired: 4 in, 4 out]
  }
  n156 = stacked-sequence {
    tunnel: w10 -> [w360]
    tunnel: w7 -> [w356]
    tunnel: w5 -> [w359]
    tunnel: "Finished" ("element") -> [w354]
    frame #0 {
      n157 = Unbundle By Name(w359) -> ("Event"=w358:refnum<event-registration>)
      n158 = Enqueue Element(queue=w356, element=w354) -> (error out=w355:errorcluster)  [unwired: 2 in, 2 out]
      n159 = property class="VI"(error in=w355, "Front Panel.Open"=FALSE ("Front Panel Window:Open")) -> ()  [unwired: 1 in, 2 out]
      n160 = Unregister For Events(event registration refnum=w358) -> ()  [unwired: 1 in, 1 out]
      "error out" <- w360
    }
  }
